vi "DMM Manual Battery Cell Measurement.vi"(8 "error in":errorcluster) -> (0 "error out":errorcluster, 2 "Measurements (Volts) All":dbl[][](array[numeric]))   [LabVIEW 2019]
panel:
  out "Measurements (Volts) ch4":dbl[](array[numeric])
  out "Measurements (Volts) ch3":dbl[](array[numeric])
  out "Measurements (Volts) ch2":dbl[](array[numeric])
  out "Measurements (Volts) ch1":dbl[](array[numeric])
  out "Measurements (Volts) ch0":dbl[](array[numeric])
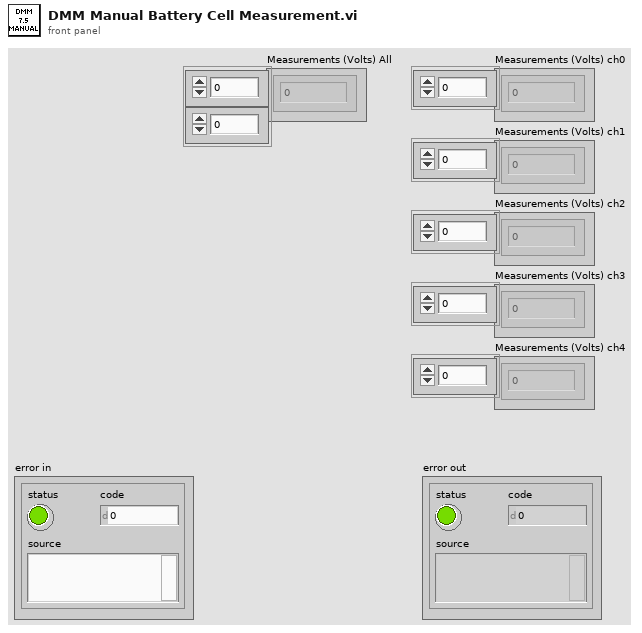
[diagram p1: front panel]
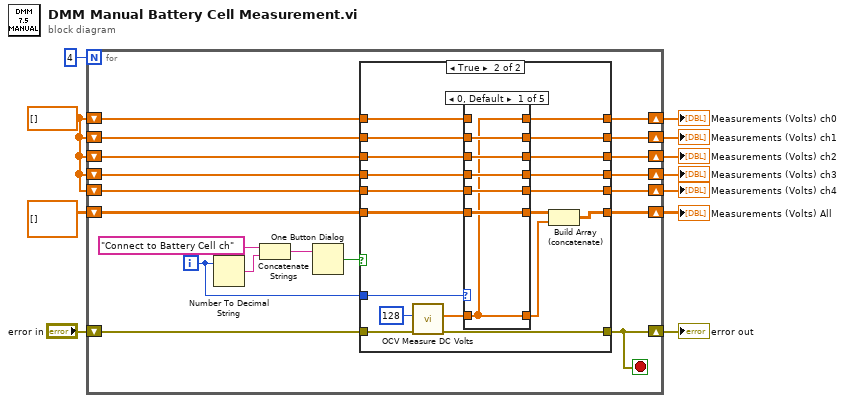
[diagram p0: block diagram]
diagram:
  w4 = dbl[] [] ("Measurements (Volts)")
  n1 = for {
    N: 4 -> [_]
    shift-right: [w25] -> w9
    shift-left: "error in" -> [w26]
    shift-right: [w23] -> w8
    shift-left: w4 -> [w22]
    shift-right: [w21] -> w7
    shift-left: w4 -> [w20]
    shift-right: [w19] -> w6
    shift-left: w4 -> [w18]
    shift-right: [w17] -> w5
    shift-left: w4 -> [w16]
    shift-right: [w15] -> w3
    shift-left: w4 -> [w14]
    shift-right: [w12] -> w1
    shift-left: dbl[][] [] ("Measurements (Volts) All") -> [w13]
    i -> [w24]
    stop <- w25 stop-if-true
    n2 = Number To Decimal String(number=w24) -> (decimal integer string=w30:string)  [unwired: 1 in]
    n3 = Concatenate Strings("Connect to Battery Cell ch" ("message"), w30) -> (w28:string)
    n4 = One Button Dialog(message=w28) -> (true=w27:bool)  [unwired: 1 in]
    n5 = case shown="True" w27 {
      tunnel: [w37 w55] -> w25
      tunnel: w26 -> [w37 w54]
      tunnel: w24 -> [_ w53]
      tunnel: [w36 w51] -> w23
      tunnel: w22 -> [w36 w50]
      tunnel: [w35 w49] -> w21
      tunnel: w20 -> [w35 w48]
      tunnel: [w34 w47] -> w19
      tunnel: w18 -> [w34 w46]
      tunnel: [w33 w45] -> w17
      tunnel: w16 -> [w33 w44]
      tunnel: [w32 w43] -> w15
      tunnel: w14 -> [w32 w42]
      tunnel: w13 -> [w31 w41]
      tunnel: [w31 w38] -> w12
      frame False {
      }
      frame True {
        n6 = call "OCV Measure DC Volts.vi"("error in (no error)"=w54, "Number of Measurements"=128) -> ("error out"=w55:errorcluster, "Measurements (Volts)"=w52:dbl[])  [unwired: 8 in]
        n7 = case shown="0, Default" w53 {
          tunnel: w52 -> [w57 w63 w69 w75 w81]
          tunnel: [w57 w68 w74 w80 w86] -> w51
          tunnel: w50 -> [_ w68 w74 w80 w86]
          tunnel: [w62 w63 w73 w79 w85] -> w49
          tunnel: w48 -> [w62 _ w73 w79 w85]
          tunnel: [w61 w67 w69 w78 w84] -> w47
          tunnel: w46 -> [w61 w67 _ w78 w84]
          tunnel: [w60 w66 w72 w75 w83] -> w45
          tunnel: w44 -> [w60 w66 w72 _ w83]
          tunnel: [w59 w65 w71 w77 w81] -> w43
          tunnel: w42 -> [w59 w65 w71 w77 _]
          tunnel: w41 -> [w58 w64 w70 w76 w82]
          tunnel: [w58 w64 w70 w76 w82] -> w40
          tunnel: [w57 w63 w69 w75 w81] -> w39
          frame 0, Default {
          }
          frame 1 {
          }
          frame 2 {
          }
          frame 3 {
          }
          frame 4 {
          }
        }
        n8 = Build Array (concatenate)(w40, w39) -> (w38:dbl[][])
      }
    }
  }
  "error out" <- w9
  "Measurements (Volts) ch0" <- w8
  "Measurements (Volts) ch1" <- w7
  "Measurements (Volts) ch2" <- w6
  "Measurements (Volts) ch3" <- w5
  "Measurements (Volts) ch4" <- w3
  "Measurements (Volts) All" <- w1
